vi "PressureSensorTest.vi"() -> ()   [LabVIEW 2013]
uses:
  <vilib>/Rock Robotics/SystemInterfaces/Typedef/FPGA_TypedefAnalogModule.ctl
  <vilib>/Rock Robotics/SystemInterfaces/AI/FPGA_AIChannel.ctl
  <vilib>/Rock Robotics/SystemInterfaces/DIO/FPGA_DIOChannel.ctl
  <vilib>/Rock Robotics/SystemInterfaces/DIO/FPGA_DIORelayChannel.ctl
  PressureSensorAction.ctl
panel:
  out "Voltage":dbl
  out "Pressure":dbl
  in  "PressureScaler":dbl=1.0
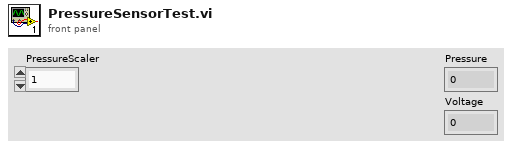
[diagram p1: front panel]
types:
  T1 = typedef "FPGA_DIORelayChannel.ctl" = enum8{"Relay 1", "Relay 2", "Relay 3", "Relay 4", "Relay 5", "Relay 6", "Relay 7", "Relay 8", "Invalid"}
  T2 = typedef "FPGA_DIOChannel.ctl" = enum8{"DIO 1", "DIO 2", "DIO 3", "DIO 4", "DIO 5", "DIO 6", "DIO 7", "DIO 8", "DIO 9", "DIO 10", "DIO 11", "DIO 12", "DIO 13", "DIO 14", "Invalid"}
  T3 = typedef "FPGA_AIChannel.ctl" = enum8{"AI 1", "AI 2", "AI 3", "AI 4", "AI 5", "AI 6", "AI 7", "AI 8", "Invalid"}
  T4 = typedef "FPGA_TypedefAnalogModule.ctl" = enum16{"Analog Module 1", "Analog Module 2"}
  T5 = typedef "WPI_AnalogChannelDevRef.ctl" = cluster{"DevStatus":errorcluster, "Analog Module":T4, "Analog Channel":T3}
  T6 = typedef "PressureSensorAction.ctl" = enum16{"Init", "ReadValue", "Disable"}
  T7 = typedef "WPI_CompressorDevRef.ctl" = cluster{"DevStatus":errorcluster, "DigitalInputDevRef":T8, "RelayDevRef":T10}
  T8 = typedef "WPI_DigitalInputDevRef.ctl" = cluster{"DevStatus":errorcluster, "DIO Channel":T2, "Digital Module":T9}
  T9 = typedef "FPGA_TypedefDigitalModule.ctl" = enum16{"Digital Module 1", "Digital Module 2"}
  T10 = typedef "WPI_RelayDevRef.ctl" = cluster{"DevStatus":errorcluster, "Relay Channel":T1, "Digital Module":T9, "Relay Direction":T11}
  T11 = typedef "WPI_RelayDirection.ctl" = enum16{"Both directions", "Forward only", "Reverse only"}
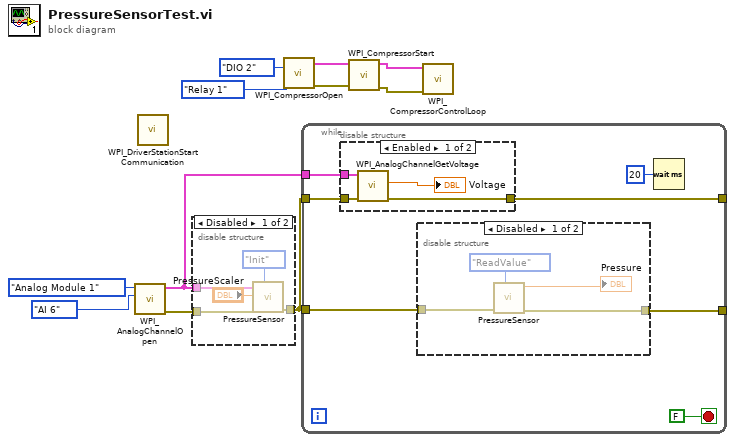
[diagram p0: block diagram]
diagram:
  n1 = call <vilib>:"WPI_AnalogChannelOpen.vi"("Analog Channel"=FPGA_AIChannel."AI 6", "Analog Module (Module 1)"=FPGA_TypedefAnalogModule."Analog Module 1") -> ("error out"=w9:errorcluster, "AIDeviceRef"=w2:T5)  [unwired: 8 in]
  n2 = call <vilib>:"WPI_DriverStationStart Communication.vi"() -> ()  [unwired: 12 in]
  n3 = disable-structure shown="Disabled" {
    disable-tunnel: w2 -> [w15 _]
    disable-tunnel: w9 -> [w14 _]
    disable-tunnel: [w12 _] -> w1
    frame Disabled {
      n4 = call "PressureSensor.vi"("Action"=PressureSensorAction."Init", "error in (no error)"=w14, "PressureScaler"="PressureScaler", "AIDeviceRef"=w15) -> ("error out"=w12:errorcluster)  [unwired: 6 in, 1 out]
    }
    frame Enabled {
    }
  }
  n5 = call <vilib>:"WPI_CompressorOpen.vi"("Pressure Switch DIO Channel"=FPGA_DIOChannel."DIO 2", "Relay Channel"=FPGA_DIORelayChannel."Relay 1") -> ("CompressorDevRef"=w8:T7, "error out"=w5:errorcluster)  [unwired: 12 in]
  n6 = while {
    tunnel: w1 -> [w22]
    tunnel: [w21] -> _
    tunnel: w2 -> [w19]
    tunnel: w1 -> [w18]
    tunnel: [w17] -> _
    stop <- FALSE stop-if-true
    n7 = disable-structure shown="Enabled" {
      disable-tunnel: w19 -> [w27 _]
      disable-tunnel: w18 -> [w26 _]
      disable-tunnel: [w25 _] -> w17
      frame Enabled {
        n8 = call <vilib>:"WPI_AnalogChannelGetVoltage.vi"("error in (no error)"=w26, "AIDeviceRef"=w27) -> ("error out"=w25:errorcluster, "Voltage"=→"Voltage":dbl)  [unwired: 7 in, 1 out]
      }
      frame Disabled {
      }
    }
    n9 = disable-structure shown="Disabled" {
      disable-tunnel: w22 -> [w30 _]
      disable-tunnel: [w29 _] -> w21
      frame Disabled {
        n10 = call "PressureSensor.vi"("Action"=PressureSensorAction."ReadValue", "error in (no error)"=w30) -> ("error out"=w29:errorcluster, "Pressure"=→"Pressure":dbl)  [unwired: 8 in]
      }
      frame Enabled {
      }
    }
    n11 = Wait (ms)(milliseconds to wait=u32 20) -> ()  [unwired: 1 out]
  }
  n12 = call <vilib>:"WPI_CompressorStart.vi"("error in (no error)"=w5, "CompressorDevRef"=w8) -> ("error out"=w6:errorcluster, "CompressorDevRef"=w7:T7)  [unwired: 8 in]
  n13 = call <vilib>:"WPI_CompressorControlLoop.vi"("error in (no error)"=w6, "CompressorDevRef"=w7) -> ()  [unwired: 10 in]
